vi "IniFileArray.vi"(8 "ErrorArray In":errorcluster[](array[cluster]), 10 "Relative Path to Plugins":path=path "") -> (0 "ErrorArray Out":errorcluster[](array[cluster]), 2 "INIFilePaths":path[](array[path]))   [LabVIEW 2014, in "Framework.lvlib"]
uses:
  Framework.lvlib
  <userlib>/NIST/NISTErrorLib/NISTErrorLib.lvlib
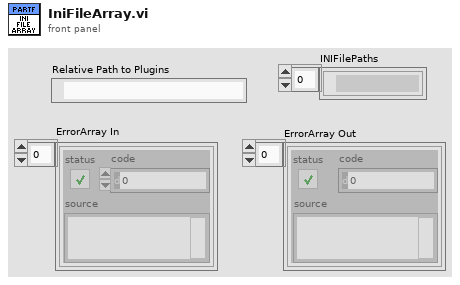
[diagram p1: front panel]
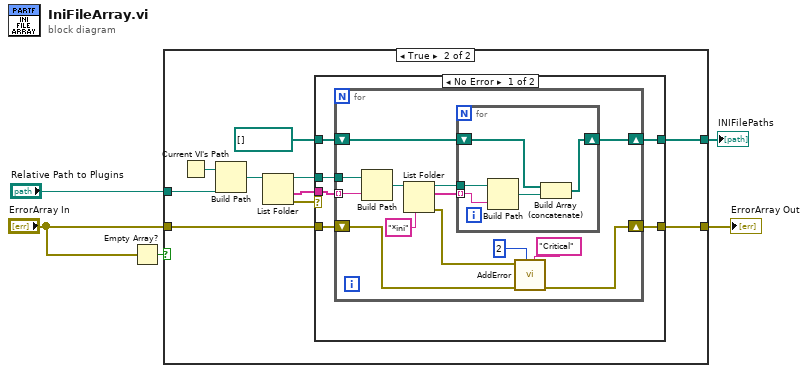
[diagram p0: block diagram]
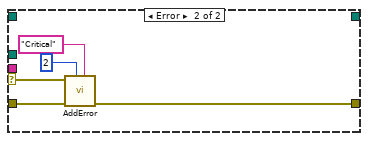
[diagram p3: hidden frame]
diagram:
  n1 = Empty Array?(array="ErrorArray In") -> (empty?=w5:bool)
  n2 = case shown="True" w5 {
    tunnel: "ErrorArray In" -> [w6 w12]
    tunnel: "Relative Path to Plugins" -> [_ w14]
    tunnel: [w6 w11] -> w2
    tunnel: [_ w7] -> w1
    frame False {
    }
    frame True {
      n3 = Current VI's Path() -> (path=w16:path)
      n4 = Build Path(base path=w16, name or relative path=w14) -> (appended path=w15:path)
      n5 = List Folder(path=w15) -> (path out=w8:path, folder names=w9:string[], error out=w13:errorcluster)  [unwired: 3 in, 1 out]
      n6 = case shown="No Error" w13 {
        selector: w13 -> [_ w44]
        tunnel: w12 -> [w19 w45]
        tunnel: [w18 w41] -> w11
        tunnel: path[] [] ("EvtINIFilePaths 2") -> [w22 _]
        tunnel: w9 -> [w21 _]
        tunnel: w8 -> [w20 _]
        tunnel: [w17 _] -> w7
        frame No Error {
          n7 = for {
            shift-right: [w28] -> w17
            shift-left: w22 -> [w29]
            tunnel: w21 -> [w31] mode=indexing
            tunnel: w20 -> [w32]
            shift-right: [w26] -> w18
            shift-left: w19 -> [w27]
            n8 = Build Path(base path=w32, name or relative path=w31) -> (appended path=w34:path)
            n9 = List Folder(path=w34, pattern="*ini") -> (path out=w30:path, filenames=w33:string[], error out=w23:errorcluster)  [unwired: 2 in, 1 out]
            n10 = for {
              tunnel: w33 -> [w38] mode=indexing
              tunnel: w30 -> [w39]
              shift-right: [w37] -> w28
              shift-left: w29 -> [w36]
              n11 = Build Path(base path=w39, name or relative path=w38) -> (appended path=w40:path)
              n12 = Build Array (concatenate)(w36, w40) -> (w37:path[])
            }
            n13 = call <userlib>:"AddError.vi"("Severity"="Critical", "Priority"=u8 2, "ErrorArray"=w27, "error in (no error)"=w23) -> ("ErrorArray"=w26:errorcluster[])  [unwired: 6 in, 1 out]
          }
        }
        frame Error {
          n14 = call <userlib>:"AddError.vi"("Severity"="Critical", "Priority"=u8 2, "ErrorArray"=w45, "error in (no error)"=w44) -> ("ErrorArray"=w41:errorcluster[])  [unwired: 6 in, 1 out]
        }
      }
    }
  }
  "ErrorArray Out" <- w2
  "INIFilePaths" <- w1
